vi "TestIOCMD.vi"(4 "QueueIOCMD":refnum<queue>, 5 "ControlInterfce":variant, 6 "ID":string, 7 "IODeviceName":string) -> ()   [LabVIEW 2020]
panel:
  out "InStart":string
  out "OutStart":string
  out "stop":bool
  out "Change Position":i32
  out "output cluster":T1
  out "DInList":string[](array[string])
  out "DOutList":string[](array[string])
  out "IO":bool
  out "Din":bool[](array[boolean])
  in  "Dout":bool[](array[boolean])
  out "CMD":T1
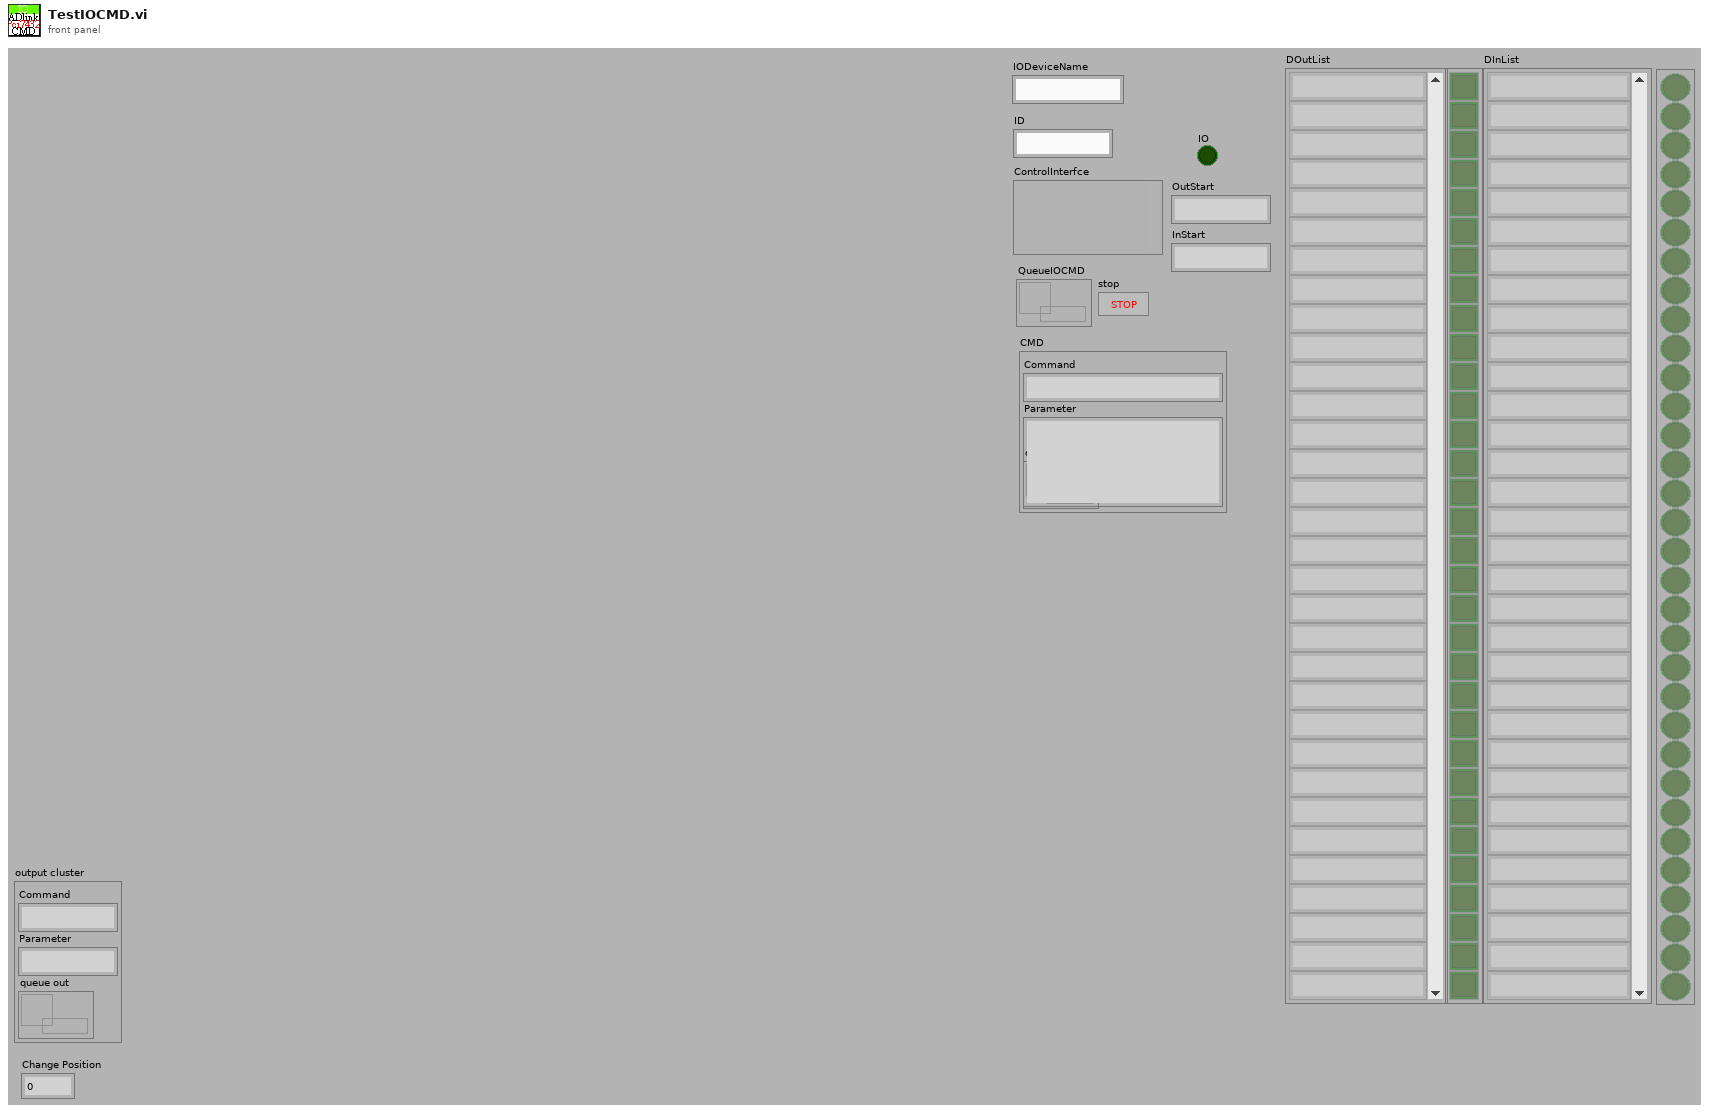
[diagram p1: front panel]
types:
  T1 = cluster{"Command":string, "Parameter":string, "queue out":refnum<queue>}
  T2 = cluster{variant, "trimmed string":string, "ID":string, "OutStart":string, "OutPorts":i32, "InStart":string, "InPorts":i32}
  T3 = cluster{"Driver":string, "CmdQueue":refnum<queue>, refnum<vi>, "Variant":variant}
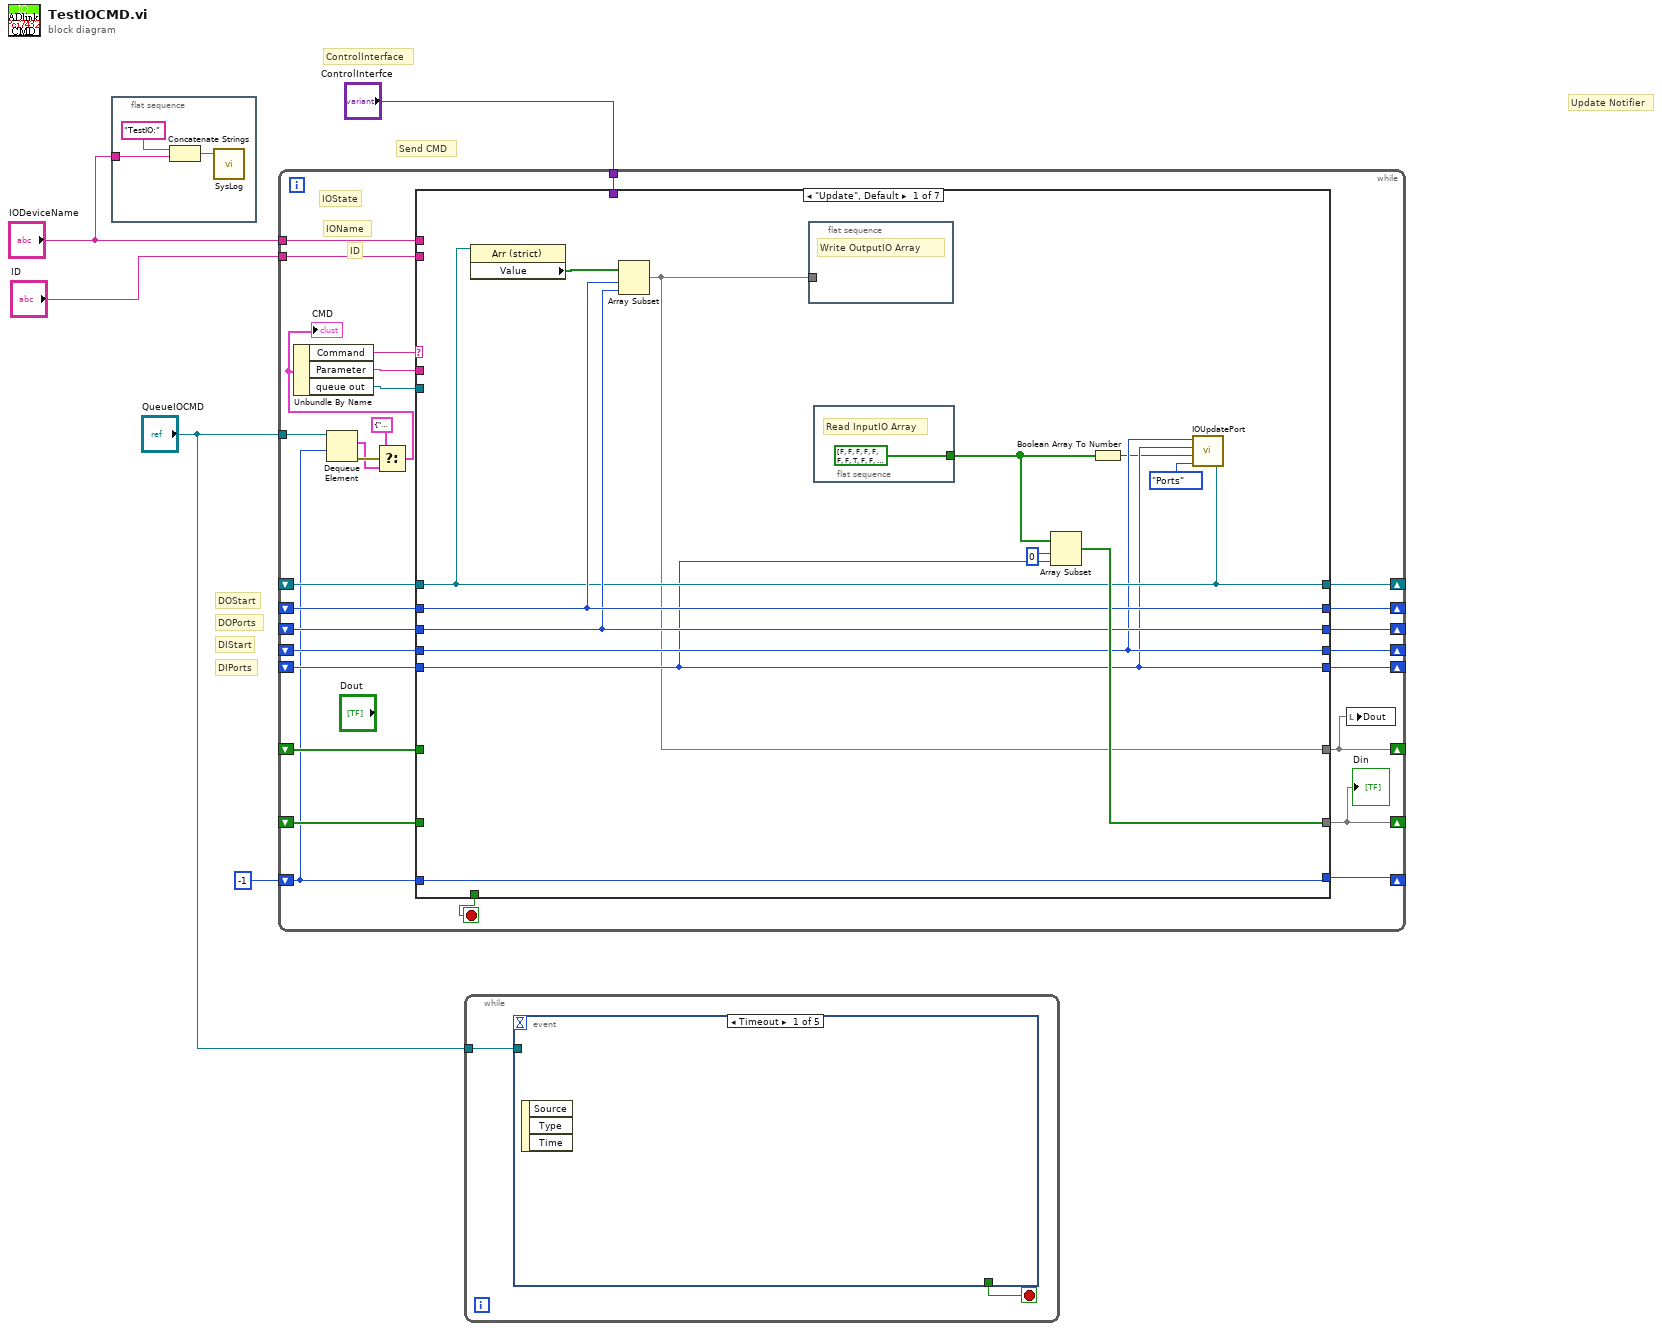
[diagram p0: block diagram]
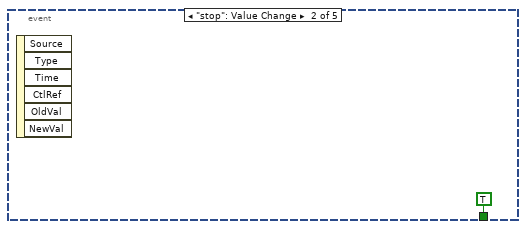
[diagram p2: hidden frame]
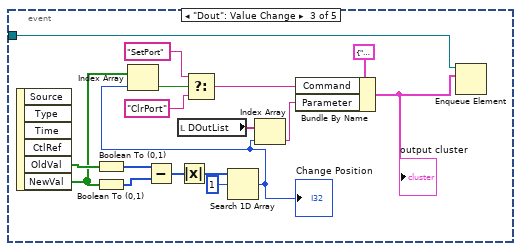
[diagram p3: hidden frame]
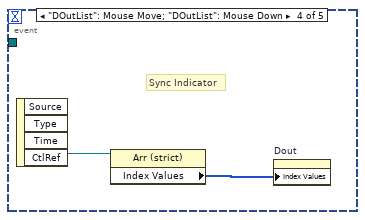
[diagram p4: hidden frame]
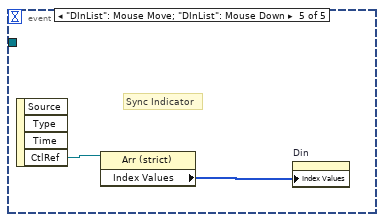
[diagram p5: hidden frame]
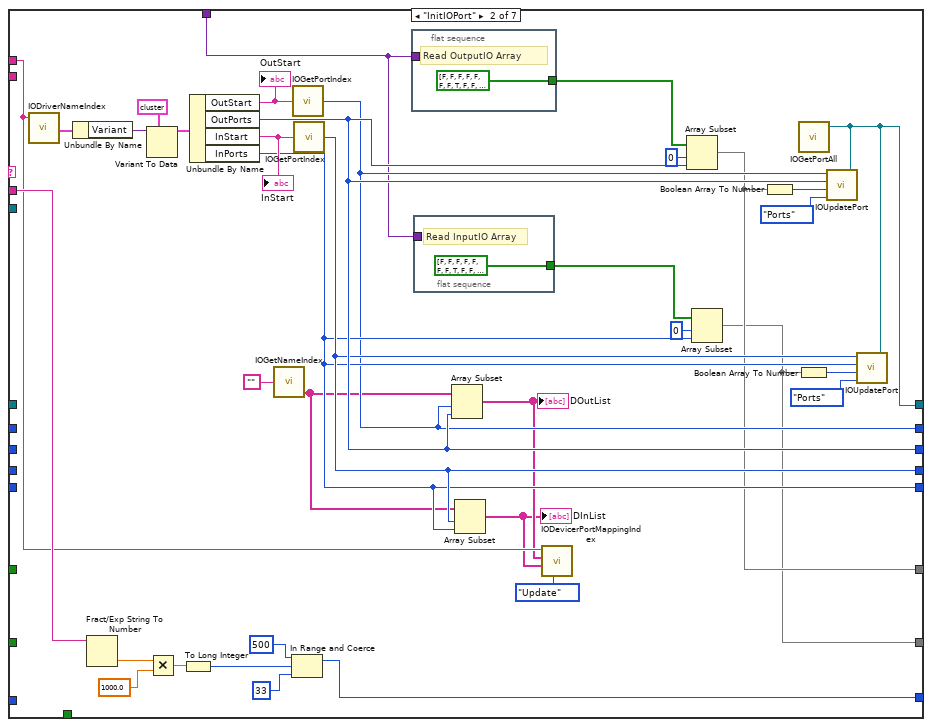
[diagram p6: hidden frame]
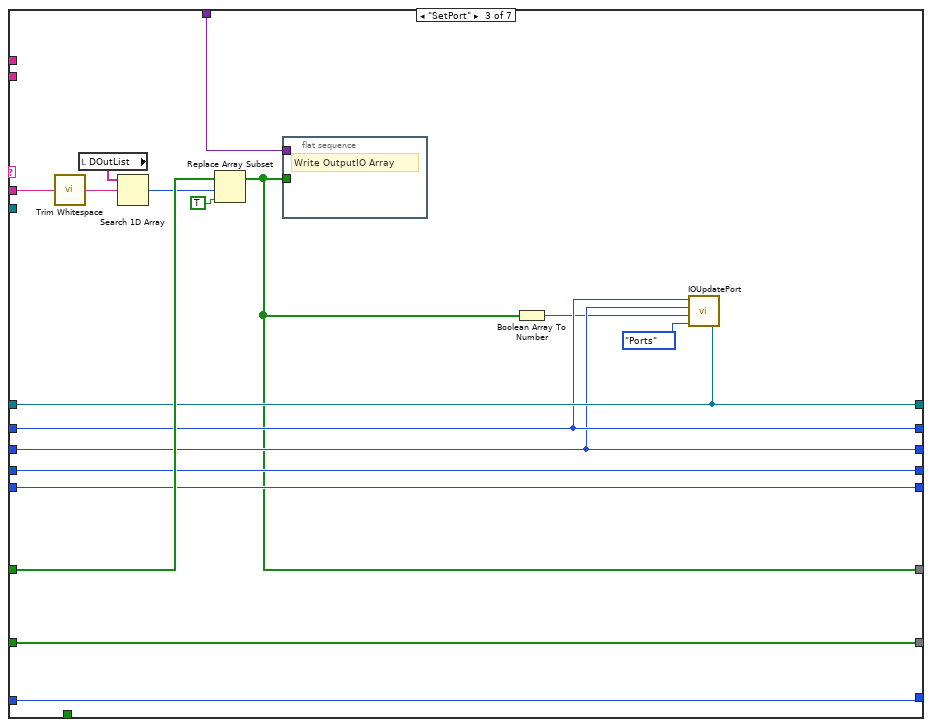
[diagram p7: hidden frame]
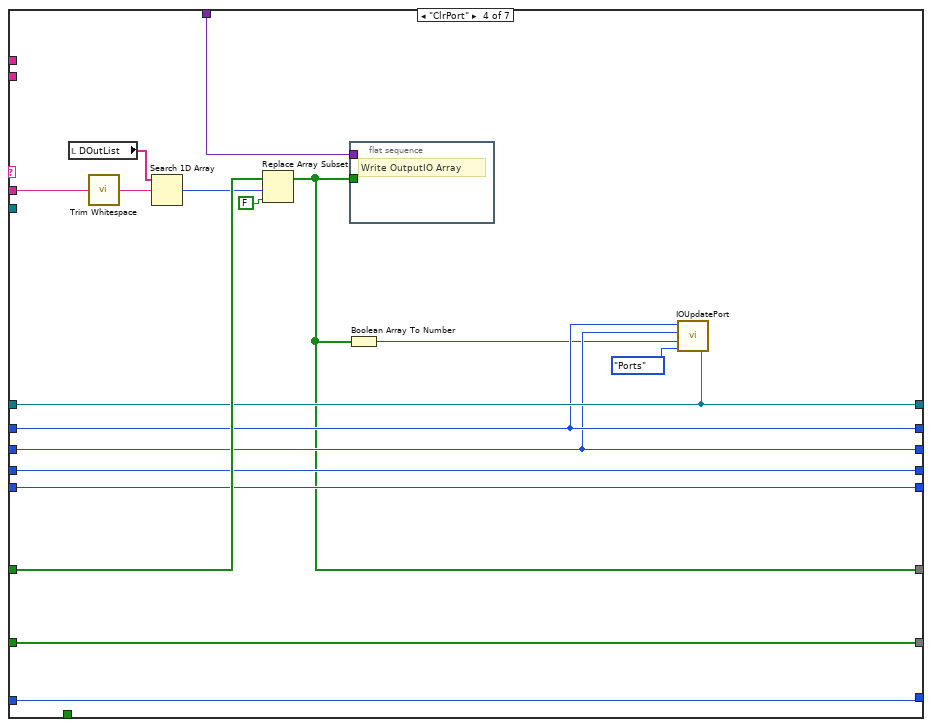
[diagram p8: hidden frame]
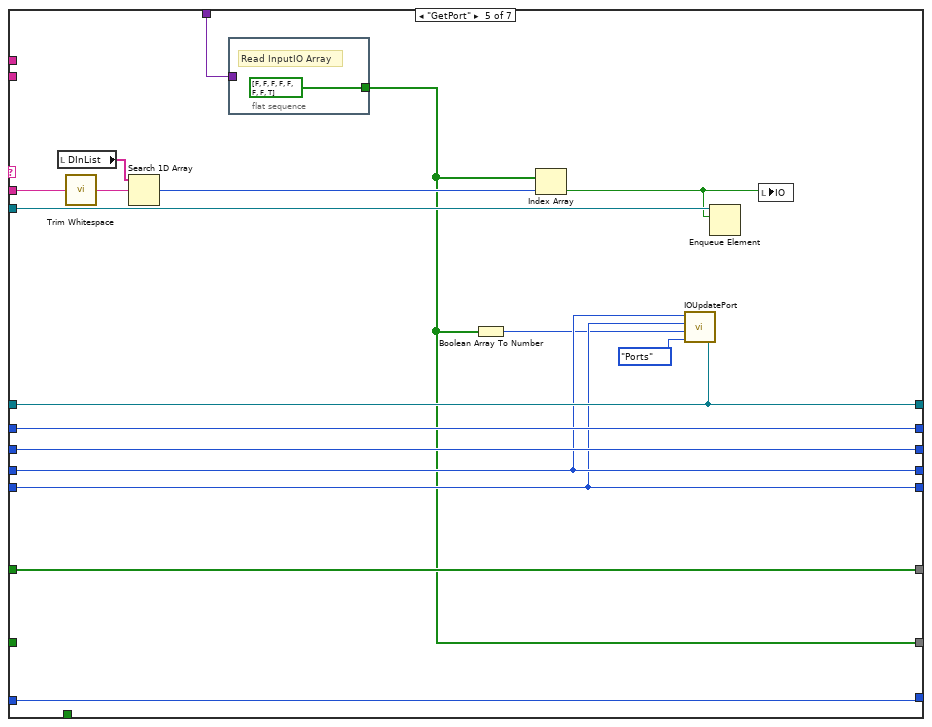
[diagram p9: hidden frame]
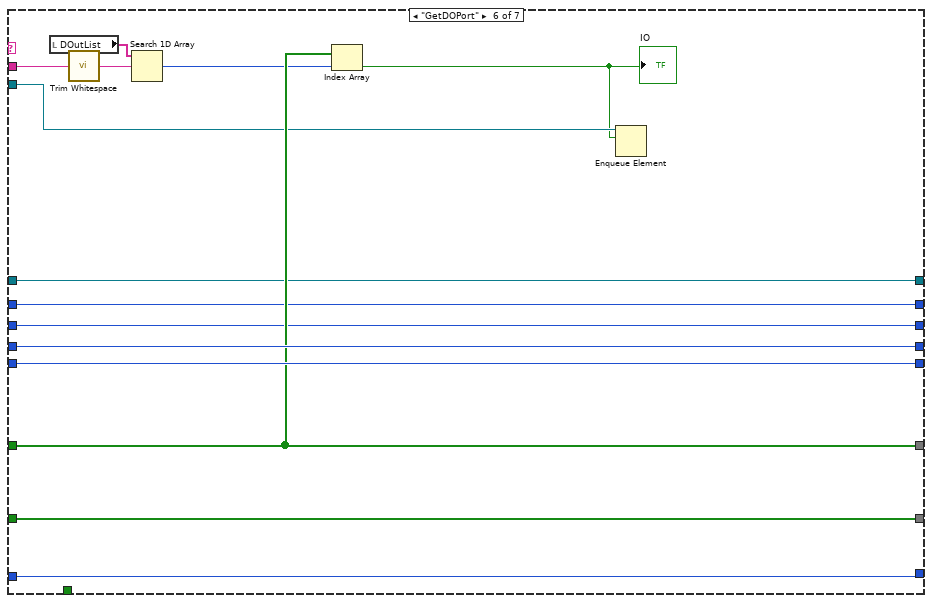
[diagram p10: hidden frame]
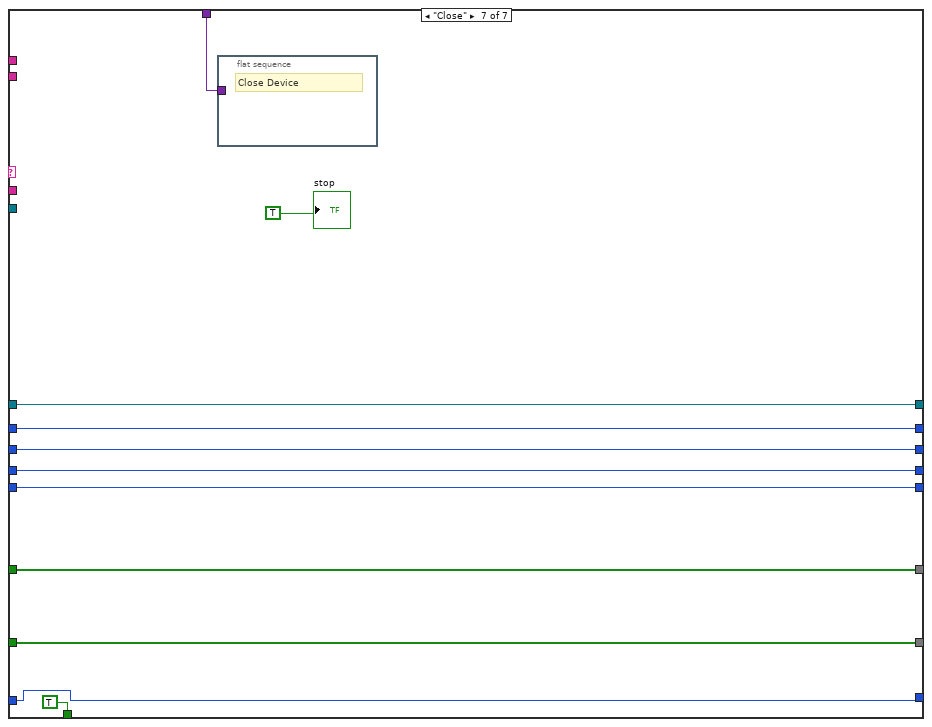
[diagram p11: hidden frame]
diagram:
  # "DIPorts"
  # "DIStart"
  # "DOPorts"
  # "DOStart"
  # "ControlInterface"
  # "Update Notifier"
  # "Send CMD"
  n1 = flat-sequence {
    tunnel: "IODeviceName" -> [w6]
    frame #0 {
      n2 = Concatenate Strings("TestIO:" ("message"), w6) -> (w8:string)
      n3 = call "SysLog.vi"("Mssage"=w8) -> ()  [unwired: 5 in]
    }
  }
  n4 = while {
    tunnel: "QueueIOCMD" -> [w36]
    tunnel: "IODeviceName" -> [w33]
    tunnel: "ID" -> [w32]
    tunnel: "ControlInterfce" -> [w30]
    shift-right: [w29] -> _
    shift-left: _ -> [w27]
    shift-right: [w14] -> _
    shift-left: _ -> [w28]
    shift-right: [w25] -> _
    shift-left: _ -> [w19]
    shift-right: [w26] -> _
    shift-left: _ -> [w20]
    shift-right: [w24] -> _
    shift-left: _ -> [w21]
    shift-right: [w23] -> _
    shift-left: _ -> [w18]
    shift-right: [w22] -> _
    shift-left: _ -> [w17]
    shift-right: [w15] -> _
    shift-left: -1 ("QueueWait") -> [w16]
    stop <- w31 stop-if-true
    # "IOState"
    # "ID"
    # "IOName"
    n5 = Dequeue Element(queue=w36, timeout in ms (-1)=w16) -> (element=w11:T1, error out=w12:errorcluster)  [unwired: 1 in, 2 out]
    n6 = Select(t=T1 {"Command"="Close", "Parameter"="", "queue out"=refnum}, s=w12, f=w11) -> (s? t:f=w10:T1)
    "CMD" <- w10
    n7 = Unbundle By Name(w10) -> ("Command"=w13:string, "Parameter"=w35:string, "queue out"=w34:refnum<queue>)
    n8 = case shown="\"Update\", Default" w13 {
      tunnel: w35 -> [_ w79 w98 w115 w132 w143 _]
      tunnel: w34 -> [_ _ _ _ w136 w147 _]
      tunnel: w33 -> [_ w53 _ _ _ _ _]
      tunnel: w32 -> [_ _ _ _ _ _ _]
      tunnel: [_ _ _ _ _ _ TRUE] -> w31
      tunnel: w30 -> [_ w61 w89 w106 w124 _ w155]
      tunnel: [w39 w58 w90 w107 w139 w151 w164] -> w14
      tunnel: [w49 w57 w104 w121 w125 w154 w163] -> w29
      tunnel: w28 -> [_ _ w103 w120 w139 w151 w164]
      tunnel: w27 -> [_ _ w104 w121 _ w154 w163]
      tunnel: [w48 w65 w93 w110 w138 w149 w161] -> w26
      tunnel: [w47 w70 w92 w109 w137 w150 w160] -> w25
      tunnel: [w42 w68 w94 w111 w129 w148 w162] -> w24
      tunnel: [w41 w67 w102 w119 w128 w153 w159] -> w23
      tunnel: [w40 w66 w101 w118 w127 w152 w158] -> w22
      tunnel: w21 -> [w42 _ w94 w111 w129 w148 w162]
      tunnel: w20 -> [w48 _ w93 w110 w138 w149 w161]
      tunnel: w19 -> [w47 _ w92 w109 w137 w150 w160]
      tunnel: w18 -> [w41 _ w102 w119 w128 w153 w159]
      tunnel: w17 -> [w40 _ w101 w118 w127 w152 w158]
      tunnel: w16 -> [w44 _ w100 w117 w135 w146 w157]
      tunnel: [w44 w72 w100 w117 w135 w146 w157] -> w15
      frame "Update", Default {
        n9 = property class="Arr (strict)"(reference=w42) -> ("Value"=w45:bool[])  [unwired: 1 in, 2 out]
        n10 = Array Subset(array=w45, index=w48, length=w47) -> (w39:bool[])
        n11 = flat-sequence {
          tunnel: w39 -> [_]
          frame #0 {
            # "Write OutputIO Array"
          }
        }
        n12 = flat-sequence {
          tunnel: [bool[] [FALSE, FALSE, FALSE, FALSE, FALSE, FALSE, FALSE, TRUE, FALSE, FALSE, FALSE, FALSE, FALSE, FALSE, FALSE, FALSE, FALSE, FALSE, FALSE, FALSE, FALSE, FALSE, FALSE, FALSE, FALSE, FALSE, FALSE, FALSE, FALSE, FALSE, FALSE, FALSE] ("Boolean array")] -> w37
          frame #0 {
            # "Read InputIO Array"
          }
        }
        n13 = Array Subset(array=w37, index=0, length=w40) -> (w49:bool[])
        n14 = Boolean Array To Number(Boolean array=w37) -> (number=w38:u32)
        n15 = call "IOUpdatePort.vi"("IORef"=w42, "OP"=enum16{"Idle", "SetPort", "ClrPort", "Ports"}."Ports", "Value"=w38, "Ports Num"=w40, "PortStart"=w41) -> ()
      }
      frame "InitIOPort" {
        n16 = call "IODriverNameIndex.vi"("IODriverName"=w53) -> ("IODataOut"=w86:T3)  [unwired: 2 in, 2 out]
        n17 = Unbundle By Name(w86) -> ("Variant"=w85:variant)
        n18 = Fract/Exp String To Number(string=w79) -> (number=w78:dbl)  [unwired: 3 in, 1 out]
        n19 = Variant To Data(type=T2 {variant, "trimmed string"="", "ID"="", "OutStart"="", "OutPorts"=0, "InStart"="", "InPorts"=0} ("output cluster"), Variant=w85) -> (data=w84:T2)  [unwired: 1 in, 1 out]
        n20 = Multiply(x=w78, y=1000.0) -> (x*y=w76:dbl)
        n21 = To Long Integer(number=w76) -> (32bit integer=w75:i32)
        n22 = Unbundle By Name(w84) -> ("OutStart"=w83:string, "OutPorts"=w70:i32, "InStart"=w82:string, "InPorts"=w66:i32)
        "OutStart" <- w83
        "InStart" <- w82
        n23 = call "IOGetNameIndex.vi"("PortName"="") -> ("PortNameList Out"=w63:string[])  [unwired: 3 in, 1 out]
        n24 = In Range and Coerce(upper limit=500, x=w75, lower limit=33) -> (coerced(x)=w72:i32)  [unwired: 1 out]
        n25 = call "IOGetPortIndex.vi"("PortName"=w83) -> ("index"=w65:i32)  [unwired: 4 in]
        n26 = call "IOGetPortIndex.vi"("PortName"=w82) -> ("index"=w67:i32)  [unwired: 4 in]
        n27 = flat-sequence {
          tunnel: w61 -> [_]
          tunnel: [bool[] [FALSE, FALSE, FALSE, FALSE, FALSE, FALSE, FALSE, TRUE, FALSE, FALSE, FALSE, FALSE, FALSE, FALSE, FALSE, FALSE, FALSE, FALSE, FALSE, FALSE, FALSE, FALSE, FALSE, FALSE, FALSE, FALSE, FALSE, FALSE, FALSE, FALSE, FALSE, FALSE] ("Boolean array")] -> w56
          frame #0 {
            # "Read OutputIO Array"
          }
        }
        n28 = flat-sequence {
          tunnel: w61 -> [_]
          tunnel: [bool[] [FALSE, FALSE, FALSE, FALSE, FALSE, FALSE, FALSE, TRUE, FALSE, FALSE, FALSE, FALSE, FALSE, FALSE, FALSE, FALSE, FALSE, FALSE, FALSE, FALSE, FALSE, FALSE, FALSE, FALSE, FALSE, FALSE, FALSE, FALSE, FALSE, FALSE, FALSE, FALSE] ("Boolean array")] -> w55
          frame #0 {
            # "Read InputIO Array"
          }
        }
        n29 = Array Subset(array=w63, index=w65, length=w70) -> (w52:string[])
        "DOutList" <- w52
        n30 = Array Subset(array=w63, index=w67, length=w66) -> (w51:string[])
        "DInList" <- w51
        n31 = call "IODevicerPortMappingIndex.vi"("OP"=enum16{"Get", "Update", "Init"}."Update", "INs"=w51, "OUTs"=w52, "Device/IO Name"=w53) -> ()  [unwired: 5 in, 3 out]
        n32 = Array Subset(array=w56, index=0, length=w70) -> (w58:bool[])
        n33 = Array Subset(array=w55, index=0, length=w66) -> (w57:bool[])
        n34 = Boolean Array To Number(Boolean array=w58) -> (number=w60:u32)
        n35 = call "IOGetPortAll.vi"() -> ("IO Ref Out"=w68:refnum<vi>)  [unwired: 4 in, 1 out]
        n36 = Boolean Array To Number(Boolean array=w57) -> (number=w59:u32)
        n37 = call "IOUpdatePort.vi"("IORef"=w68, "OP"=enum16{"Idle", "SetPort", "ClrPort", "Ports"}."Ports", "Value"=w60, "Ports Num"=w70, "PortStart"=w65) -> ()
        n38 = call "IOUpdatePort.vi"("IORef"=w68, "OP"=enum16{"Idle", "SetPort", "ClrPort", "Ports"}."Ports", "Value"=w59, "Ports Num"=w66, "PortStart"=w67) -> ()
      }
      frame "SetPort" {
        n39 = call <vilib>:"Trim Whitespace.vi"("string"=w98) -> ("trimmed string"=w97:string)  [unwired: 1 in]
        n40 = local read "DOutList"() -> (w99:string[])
        n41 = Search 1D Array(1D array=w99, element=w97) -> (index of element=w96:i32)  [unwired: 1 in]
        n42 = Replace Array Subset(array=w103, new element=TRUE ("new element/subarray"), index=w96) -> (w90:bool[])
        n43 = flat-sequence {
          tunnel: w90 -> [_]
          tunnel: w89 -> [_]
          frame #0 {
            # "Write OutputIO Array"
          }
        }
        n44 = Boolean Array To Number(Boolean array=w90) -> (number=w91:u32)
        n45 = call "IOUpdatePort.vi"("IORef"=w94, "OP"=enum16{"Idle", "SetPort", "ClrPort", "Ports"}."Ports", "Value"=w91, "Ports Num"=w92, "PortStart"=w93) -> ()
      }
      frame "ClrPort" {
        n46 = local read "DOutList"() -> (w114:string[])
        n47 = call <vilib>:"Trim Whitespace.vi"("string"=w115) -> ("trimmed string"=w116:string)  [unwired: 1 in]
        n48 = Search 1D Array(1D array=w114, element=w116) -> (index of element=w113:i32)  [unwired: 1 in]
        n49 = Replace Array Subset(array=w120, new element=FALSE ("new element/subarray"), index=w113) -> (w107:bool[])
        n50 = Boolean Array To Number(Boolean array=w107) -> (number=w108:u32)
        n51 = flat-sequence {
          tunnel: w107 -> [_]
          tunnel: w106 -> [_]
          frame #0 {
            # "Write OutputIO Array"
          }
        }
        n52 = call "IOUpdatePort.vi"("IORef"=w111, "OP"=enum16{"Idle", "SetPort", "ClrPort", "Ports"}."Ports", "Value"=w108, "Ports Num"=w109, "PortStart"=w110) -> ()
      }
      frame "GetPort" {
        n53 = local read "DInList"() -> (w131:string[])
        n54 = call <vilib>:"Trim Whitespace.vi"("string"=w132) -> ("trimmed string"=w134:string)  [unwired: 1 in]
        n55 = Search 1D Array(1D array=w131, element=w134) -> (index of element=w133:i32)  [unwired: 1 in]
        n56 = flat-sequence {
          tunnel: [bool[] [FALSE, FALSE, FALSE, FALSE, FALSE, FALSE, FALSE, TRUE] ("Boolean array")] -> w125
          tunnel: w124 -> [_]
          frame #0 {
            # "Read InputIO Array"
          }
        }
        n57 = Boolean Array To Number(Boolean array=w125) -> (number=w126:u32)
        n58 = Index Array(array=w125, index=w133) -> (element=w123:bool)
        n59 = call "IOUpdatePort.vi"("IORef"=w129, "OP"=enum16{"Idle", "SetPort", "ClrPort", "Ports"}."Ports", "Value"=w126, "Ports Num"=w127, "PortStart"=w128) -> ()
        n60 = Enqueue Element(queue=w136, element=w123) -> ()  [unwired: 2 in, 3 out]
        n61 = local write "IO"(w123) -> ()
      }
      frame "GetDOPort" {
        n62 = local read "DOutList"() -> (w142:string[])
        n63 = call <vilib>:"Trim Whitespace.vi"("string"=w143) -> ("trimmed string"=w145:string)  [unwired: 1 in]
        n64 = Search 1D Array(1D array=w142, element=w145) -> (index of element=w144:i32)  [unwired: 1 in]
        n65 = Index Array(array=w151, index=w144) -> (element=w141:bool)
        "IO" <- w141
        n66 = Enqueue Element(queue=w147, element=w141) -> ()  [unwired: 2 in, 3 out]
      }
      frame "Close" {
        n67 = flat-sequence {
          tunnel: w155 -> [_]
          frame #0 {
            # "Close Device"
          }
        }
        "stop" <- TRUE
      }
    }
    "Din" <- w29
    n68 = local write "Dout"(w14) -> ()
  }
  n69 = while {
    tunnel: "QueueIOCMD" -> [w167]
    stop <- w166 stop-if-true
    n70 = event shown="[0] Timeout" {
      selector: _ -> [_ _ _ _ _]
      dyn-events: _ -> [_ _ _ _ _]
      timeout: _ -> [_ _ _ _ _]
      tunnel: [_ TRUE _ _ _] -> w166
      tunnel: w167 -> [_ _ w173 _ _]
      event Timeout {
        n71 = event-data() -> ()  [unwired: 1 in, 3 out]
      }
      event "stop": Value Change {
        n72 = event-data() -> ()  [unwired: 1 in, 6 out]
      }
      event "Dout": Value Change {
        n73 = event-data() -> ("OldVal"=w185:bool[], "NewVal"=w179:bool[])  [unwired: 1 in, 4 out]
        n74 = Boolean To (0,1)(Boolean=w185) -> (0, 1=w181:i16[])
        n75 = Boolean To (0,1)(Boolean=w179) -> (0, 1=w180:i16[])
        n76 = Subtract(x=w181, y=w180) -> (x-y=w184:i16[])
        n77 = local read "DOutList"() -> (w170:string[])
        n78 = Absolute Value(x=w184) -> (abs(x)=w183:i16[])
        n79 = Search 1D Array(1D array=w183, element=i16 1) -> (index of element=w171:i32)  [unwired: 1 in]
        "Change Position" <- w171
        n80 = Index Array(array=w179, index=w171) -> (element=w177:bool)
        n81 = Select(t="SetPort", s=w177, f="ClrPort") -> (s? t:f=w174:string)
        n82 = Index Array(array=w170, index=w171) -> (element=w169:string)
        n83 = Bundle By Name(cluster=T1 {"Command"="", "Parameter"="", "queue out"=refnum} ("element"), "Command"=w174, "Parameter"=w169) -> (w172:T1)
        "output cluster" <- w172
        n84 = Enqueue Element(queue=w173, element=w172) -> ()  [unwired: 2 in, 3 out]
      }
      event "DOutList": Mouse Move; "DOutList": Mouse Down {
        # "Sync Indicator"
        n85 = event-data() -> ("CtlRef"=w187:refnum<vi>)  [unwired: 1 in, 3 out]
        n86 = property class="Arr (strict)"(reference=w187) -> ("Index Values"=w186:u32[])  [unwired: 1 in, 2 out]
        n87 = property on="Dout" class="Arr (strict)"("Index Values"=w186) -> ()  [unwired: 2 in, 2 out]
      }
      event "DInList": Mouse Move; "DInList": Mouse Down {
        # "Sync Indicator"
        n88 = event-data() -> ("CtlRef"=w189:refnum<vi>)  [unwired: 1 in, 3 out]
        n89 = property class="Arr (strict)"(reference=w189) -> ("Index Values"=w188:u32[])  [unwired: 1 in, 2 out]
        n90 = property on="Din" class="Arr (strict)"("Index Values"=w188) -> ()  [unwired: 2 in, 2 out]
      }
    }
  }
